vi "Convert I16x4 to U64.vi"(2 "Input Data":i16[](array[numeric])=[0, 0, 0, 0]) -> (16 "U64":u64)   [LabVIEW 2012]
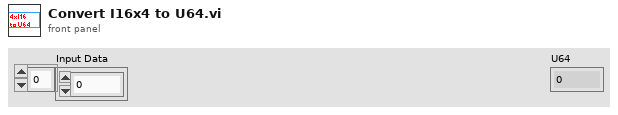
[diagram p1: front panel]
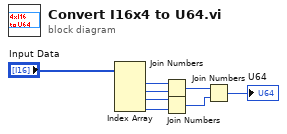
[diagram p0: block diagram]
diagram:
  n1 = Index Array(array="Input Data") -> (element #1=w6:i16, element #2=w7:i16, element #3=w5:i16, element #4=w4:i16)  [unwired: 4 in]
  n2 = Join Numbers(hi=w6, lo=w7) -> ((hi.lo)=w3:u32)
  n3 = Join Numbers(hi=w5, lo=w4) -> ((hi.lo)=w2:u32)
  n4 = Join Numbers(hi=w3, lo=w2) -> ((hi.lo)=→"U64":u64)
